vi "SENS_CORR_COLL_GUID_ADAP_DEL.vi"(0 "VISA IN":refnum<visa-resource-name>, 1 "Adapter":i32, 2 "Adapter Delay":i32, 3 "Waveguide Phae":i32, 4 "Waveguide Delay":i32, 5 "error in":errorcluster, 7 "Channel":i32=1) -> (14 "VISA Out":refnum<visa-resource-name>, 19 "error out":errorcluster)   [LabVIEW 2018, in "PNA-X.lvlib"]
doc: "SENSe<cnum>:CORRection:COLLect:GUIDed:ADAPter<n>:DELay <coax>, [w phase, \nwdelay] \n(Write-only) Specifies the adapter delay. and optionally waveguide delay and optional phase offset \n(degrees) of adapter <n>. \nParameters \n<cnum> Any existing channel number. If unspecified, value is set to 1 \n<n> Adapter index number that was returned from \nSENS:CORR:COLL:GUID:ADAP:CREate? \n<coax> Delay value of coax adapter <n> in seconds. If the adapter has no coax \nconnector, enter 0. \n<wphase> Waveguide phase offset in degrees. If the adapter has no waveguide connector, \ndo not enter a value. \n<wdelay> Waveguide delay in seconds. If the adapter has no waveguide connector, do not \nenter a value. \nExamples See example using this command. \nDefault Not Applicable"
uses:
  PNA-X.lvlib
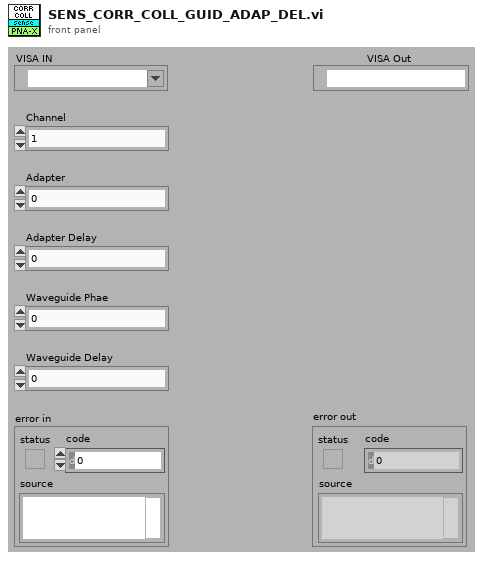
[diagram p1: front panel]
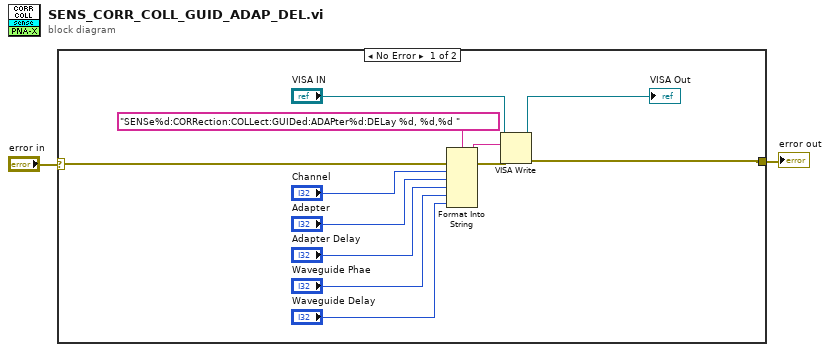
[diagram p0: block diagram]
diagram:
  n1 = case shown="No Error" "error in" {
    selector: "error in" -> [w14 w15]
    tunnel: [w9 w15] -> w1
    frame No Error {
      n2 = Format Into String(format string="SENSe%d:CORRection:COLLect:GUIDed:ADAPter%d:DELay %d, %d,%d " ("Cmdline"), error in=w14, "Channel", "Adapter", "Adapter Delay", "Waveguide Phae", "Waveguide Delay") -> (resulting string=w12:string, error out=w13:errorcluster)  [unwired: 1 in]
      n3 = VISA Write(VISA resource name="VISA IN", write buffer=w12, error in (no error)=w13) -> (VISA resource name out=→"VISA Out":refnum<visa-resource-name>, error out=w9:errorcluster)  [unwired: 1 out]
    }
    frame Error {
    }
  }
  "error out" <- w1
